vi "from string array.vi"(8 "error in (no error)":errorcluster, 9 "String Array":string[][](array[string]), 10 "version":string, 11 "module configuration in":refnum<class "Daqmx Module configuration.lvclass">) -> (0 "error out":errorcluster, 3 "module configuration out":refnum<class "Daqmx Module configuration.lvclass">)   [LabVIEW 2015, in "DAQmx Module Configuration.lvclass"]
uses:
  Daqmx Module configuration.lvclass
  Line.ctl
  <vilib>/NI/Tag Bus Module Framework/channel/TBM channel.lvclass
  Measurement Type.ctl
  Parameters.ctl
  <vilib>/NI/Tag Bus/tag/Data Type.ctl
  <vilib>/NI/Tag Bus Module Framework/channel/channel classification.ctl
  Daqmx Module configuration.lvclass/Daqmx Module configuration.ctl
  <vilib>/NI/Tag Bus/tag/tag descriptor.lvclass
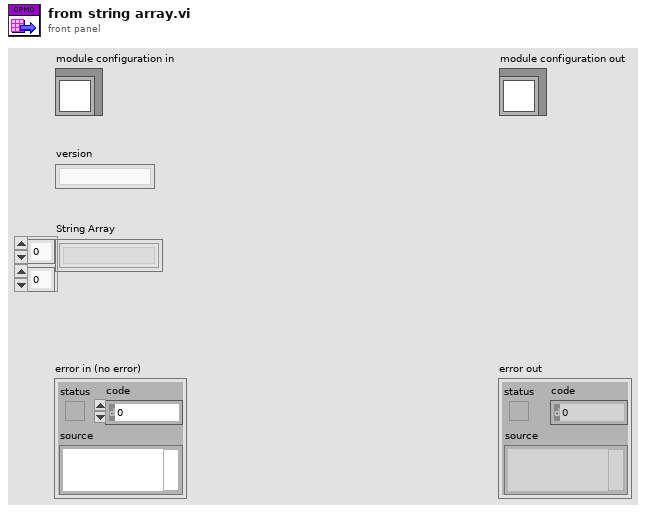
[diagram p1: front panel]
types:
  T1 = typedef "DAQmx Module Configuration.lvclass/Line.ctl" = cluster{"Channel Array":refnum<class "TBM channel.lvclass">[], "Physical Channel":string, "Measurement Type":T2, "Parameters":T3}
  T2 = typedef "DAQmx Module Configuration.lvclass/Measurement Type.ctl" = enum16{"Digital Input", "Digital Output", "Voltage Input", "Voltage Output", "Current Input", "Current Output", "RTD", "Thermocouple", "Strain", "PWM"}
  T3 = typedef "DAQmx Module Configuration.lvclass/Parameters.ctl" = cluster{"Digital Config":cluster{"Invert Lines?":bool}, "Voltage Config":cluster{"Maximum Value (V)":dbl, "Minimum Value (V)":dbl, "in terminal configuration (V)":i32, "out terminal configuration (V)":i32}, "Current Config":cluster{"Maximum Value (A)":dbl, "Minimum Value (A)":dbl, "shunt resistor location":i32, "input terminal configuration (C)":i32, "external shunt resistor value":dbl}, "RTD Config":cluster{"Maximum Value (°C)":dbl, "Minimum Value (°C)":dbl, "resistance configuration":i32, "r0":dbl, "current excitation value":dbl, "rtd type":i32, "current excitation source":i32}, "Thermocouple Config":cluster{"Minimum Value (C)":dbl, "Maximum Value (C)":dbl, "thermocouple type":i32, "cjc source":i32, "cjc value":dbl}, "Strain Config":cluster{"Maximum Value":dbl, "Minimum Value":dbl, "bridge information":cluster{"strain configuration":i32, "lead wire resistance":dbl, "initial bridge voltage":dbl, "voltage excitation source":i32, "voltage excitation value":dbl}, "strain gage information":cluster{"gage factor":dbl, "nominal gage resistance":dbl, "poisson ratio":dbl}}, "PWM Config":cluster{"Idle State":bool}}
  T4 = typedef "TBM channel.lvclass/channel classification.ctl" = enum16{"input data", "output data", "processing parameter", "processing result"}
  T5 = typedef "tag bus.lvlib/tag descriptor.lvclass/Data Type.ctl" = enum16{"Double", "Single", "I64", "I32", "I16", "I8", "U64", "U32", "U16", "U8", "Boolean", "String", "Array of Double", "Array of Single", "Array of I64", "Array of I32", "Array of I16", "Array of I8", "Array of U64", "Array of U32", "Array of U16", "Array of U8", "Array of Boolean", "Array of String"}
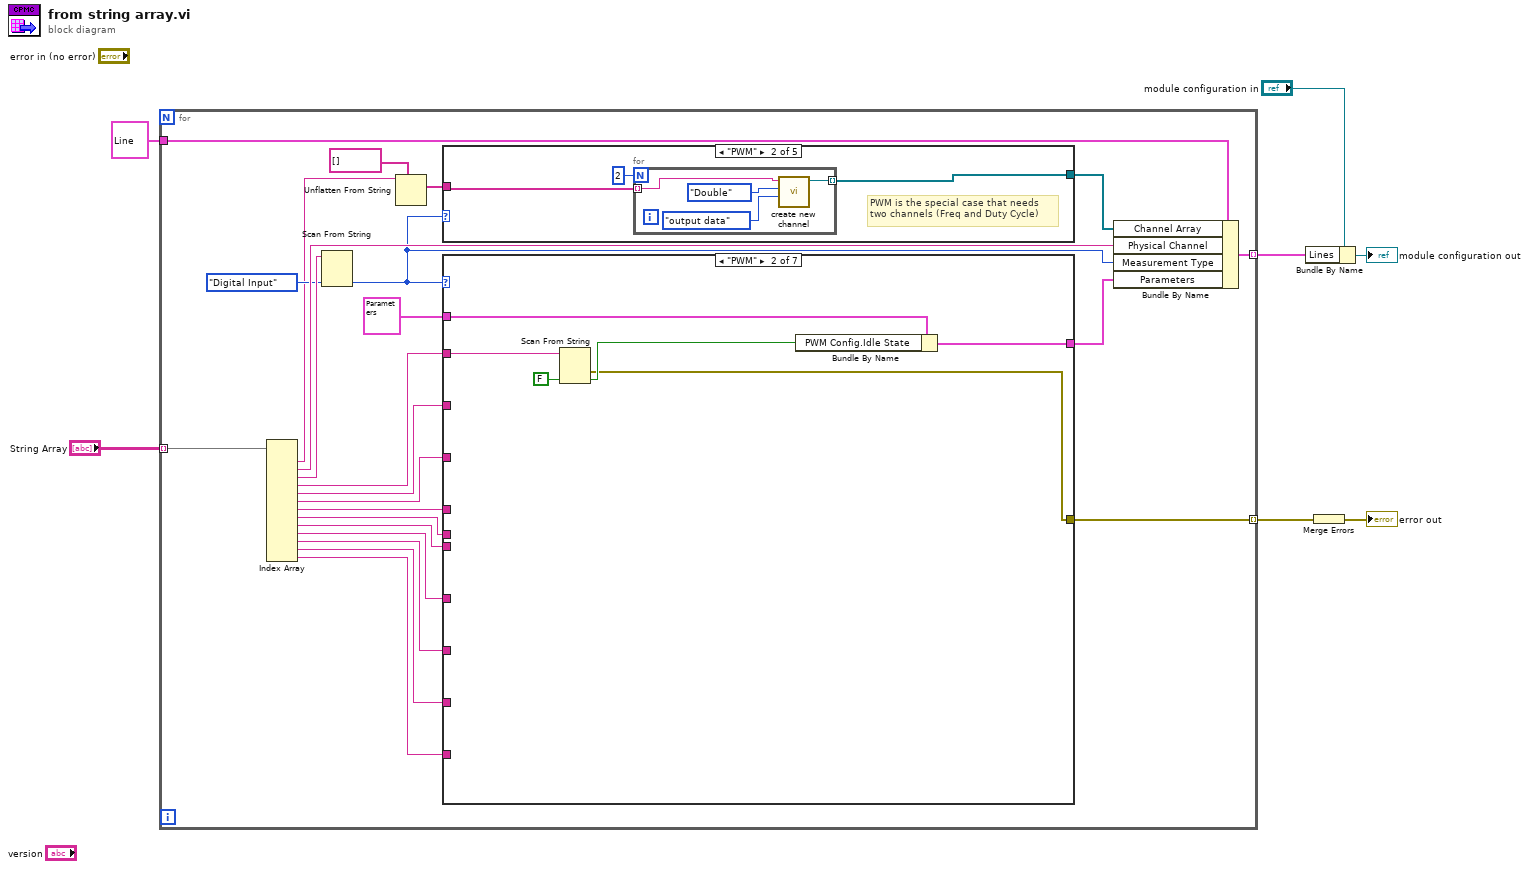
[diagram p0: block diagram]
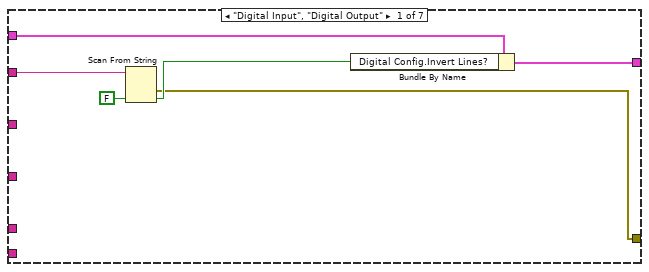
[diagram p2: hidden frame]
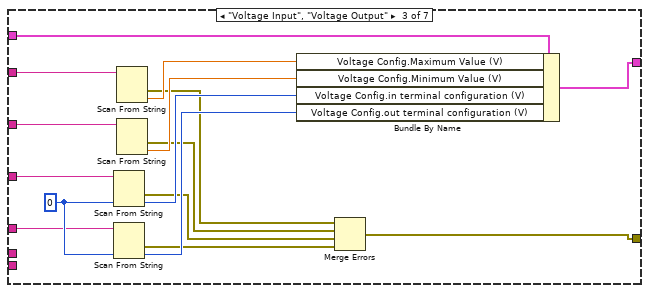
[diagram p3: hidden frame]
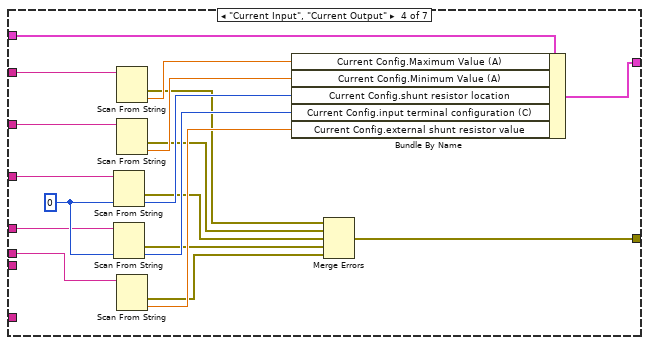
[diagram p4: hidden frame]
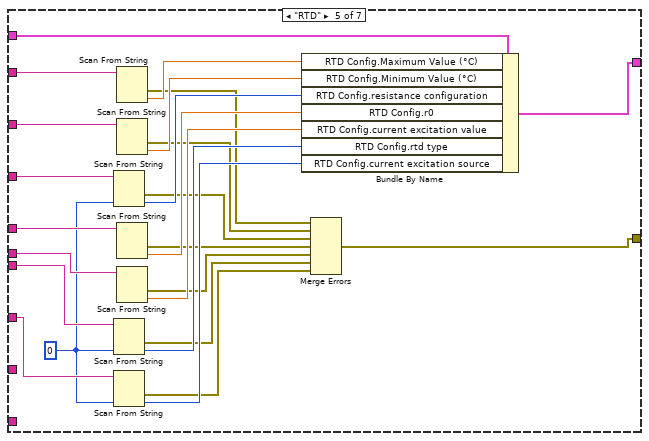
[diagram p5: hidden frame]
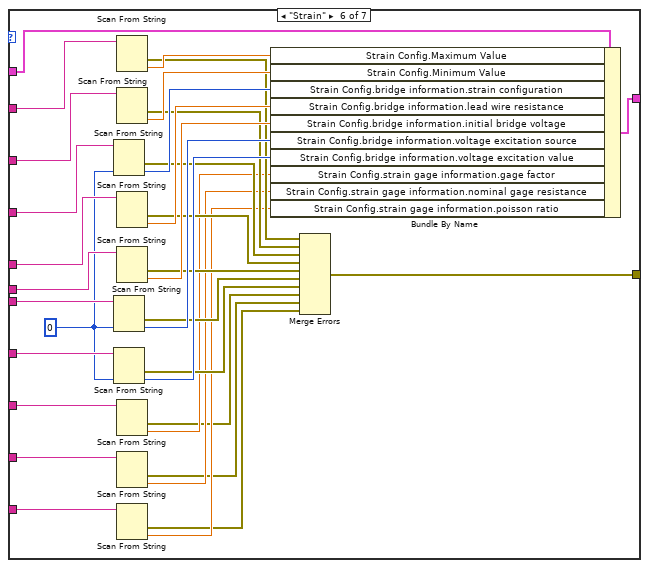
[diagram p6: hidden frame]
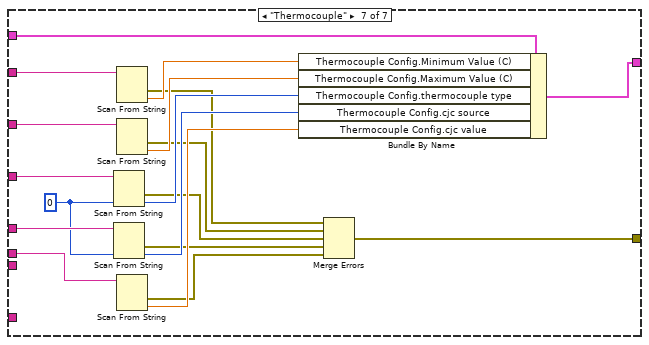
[diagram p7: hidden frame]
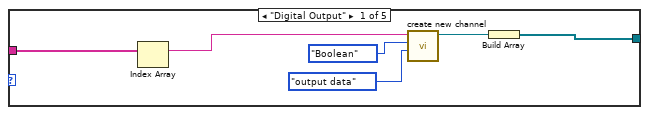
[diagram p8: hidden frame]
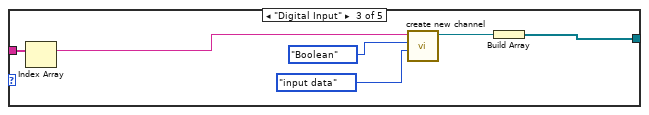
[diagram p9: hidden frame]
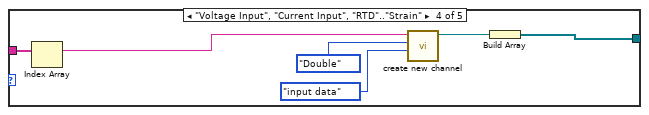
[diagram p10: hidden frame]
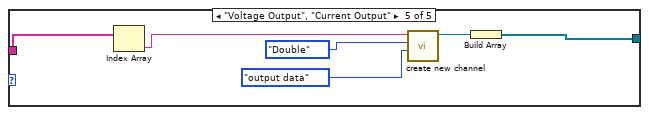
[diagram p11: hidden frame]
diagram:
  n1 = for {
    tunnel: "String Array" -> [w29] mode=indexing
    tunnel: T1 {"Channel Array"=[], "Physical Channel"="", "Measurement Type"=enum."Digital Input", "Parameters"={"Digital Config"={"Invert Lines?"=FALSE}, "Voltage Config"={"Maximum Value (V)"=5.0, "Minimum Value (V)"=-5.0, "in terminal configuration (V)"=-1, "out terminal configuration (V)"=-1}, "Current Config"={"Maximum Value (A)"=0.02, "Minimum Value (A)"=0.0, "shunt resistor location"=-1, "input terminal configuration (C)"=-1, "external shunt resistor value"=249.0}, "RTD Config"={"Maximum Value (°C)"=100.0, "Minimum Value (°C)"=0.0, "resistance configuration"=2, "r0"=100.0, "current excitation value"=0.0025, "rtd type"=10137, "current excitation source"=10167}, "Thermocouple Config"={"Minimum Value (C)"=0.0, "Maximum Value (C)"=100.0, "thermocouple type"=10072, "cjc source"=10116, "cjc value"=25.0}, "Strain Config"={"Maximum Value"=0.001, "Minimum Value"=-0.001, "bridge information"={"strain configuration"=10183, "lead wire resistance"=0.0, "initial bridge voltage"=0.0, "voltage excitation source"=10200, "voltage excitation value"=2.5}, "strain gage information"={"gage factor"=2.0, "nominal gage resistance"=350.0, "poisson ratio"=0.3}}, "PWM Config"={"Idle State"=FALSE}}} ("Line") -> [w31]
    tunnel: [w30] -> w4 mode=indexing
    tunnel: [w14] -> w2 mode=indexing
    n2 = Index Array(array=w29) -> (element #1=w9:string, element #2=w28:string, element #3=w27:string, element #4=w21:string, element #5=w20:string, element #6=w19:string, element #7=w18:string, element #8=w17:string, element #9=w16:string, element #10=w15:string, element #11=w13:string, element #12=w12:string, element #13=w11:string)  [unwired: 13 in]
    n3 = Scan From String(input string=w27, default 1=Measurement_Type."Digital Input" ("Measurement Type")) -> (output 1=w22:T2)  [unwired: 3 in, 3 out]
    n4 = Unflatten From String(type=string[] [], binary string=w9) -> (value=w8:string[])  [unwired: 3 in, 2 out]
    n5 = case shown="\"PWM\"" w22 {
      tunnel: w8 -> [w162 w164 w175 w181 w187]
      tunnel: [w158 w165 w171 w177 w183] -> w26
      frame "Digital Output" {
        n6 = Index Array(array=w162) -> (element=w157:string)  [unwired: 1 in]
        n7 = call <vilib>:"create new channel.vi"("channel classification"=channel_classification."output data", "data type"=Data_Type."Boolean", "channel name"=w157) -> ("channel"=w159:refnum<class "TBM channel.lvclass">)  [unwired: 8 in]
        n8 = Build Array(w159) -> (w158:refnum<class "TBM channel.lvclass">[])
      }
      frame "PWM" {
        # "PWM is the special case that needs\ntwo channels (Freq and Duty Cycle)"
        n9 = for {
          N: 2 -> [_]
          tunnel: [w167] -> w165 mode=indexing
          tunnel: w164 -> [w166] mode=indexing
          n10 = call <vilib>:"create new channel.vi"("channel classification"=channel_classification."output data", "data type"=Data_Type."Double", "channel name"=w166) -> ("channel"=w167:refnum<class "TBM channel.lvclass">)  [unwired: 8 in]
        }
      }
      frame "Digital Input" {
        n11 = Index Array(array=w175) -> (element=w170:string)  [unwired: 1 in]
        n12 = call <vilib>:"create new channel.vi"("channel classification"=channel_classification."input data", "data type"=Data_Type."Boolean", "channel name"=w170) -> ("channel"=w172:refnum<class "TBM channel.lvclass">)  [unwired: 8 in]
        n13 = Build Array(w172) -> (w171:refnum<class "TBM channel.lvclass">[])
      }
      frame "Voltage Input", "Current Input", "RTD".."Strain" {
        n14 = Index Array(array=w181) -> (element=w176:string)  [unwired: 1 in]
        n15 = call <vilib>:"create new channel.vi"("channel classification"=channel_classification."input data", "data type"=Data_Type."Double", "channel name"=w176) -> ("channel"=w178:refnum<class "TBM channel.lvclass">)  [unwired: 8 in]
        n16 = Build Array(w178) -> (w177:refnum<class "TBM channel.lvclass">[])
      }
      frame "Voltage Output", "Current Output" {
        n17 = Index Array(array=w187) -> (element=w182:string)  [unwired: 1 in]
        n18 = call <vilib>:"create new channel.vi"("channel classification"=channel_classification."output data", "data type"=Data_Type."Double", "channel name"=w182) -> ("channel"=w184:refnum<class "TBM channel.lvclass">)  [unwired: 8 in]
        n19 = Build Array(w184) -> (w183:refnum<class "TBM channel.lvclass">[])
      }
    }
    n20 = case shown="\"PWM\"" w22 {
      tunnel: T3 {"Digital Config"={"Invert Lines?"=FALSE}, "Voltage Config"={"Maximum Value (V)"=5.0, "Minimum Value (V)"=-5.0, "in terminal configuration (V)"=-1, "out terminal configuration (V)"=-1}, "Current Config"={"Maximum Value (A)"=0.02, "Minimum Value (A)"=0.0, "shunt resistor location"=-1, "input terminal configuration (C)"=-1, "external shunt resistor value"=249.0}, "RTD Config"={"Maximum Value (°C)"=100.0, "Minimum Value (°C)"=0.0, "resistance configuration"=2, "r0"=100.0, "current excitation value"=0.0025, "rtd type"=10137, "current excitation source"=10167}, "Thermocouple Config"={"Minimum Value (C)"=0.0, "Maximum Value (C)"=100.0, "thermocouple type"=10072, "cjc source"=10116, "cjc value"=25.0}, "Strain Config"={"Maximum Value"=0.001, "Minimum Value"=-0.001, "bridge information"={"strain configuration"=10183, "lead wire resistance"=0.0, "initial bridge voltage"=0.0, "voltage excitation source"=10200, "voltage excitation value"=2.5}, "strain gage information"={"gage factor"=2.0, "nominal gage resistance"=350.0, "poisson ratio"=0.3}}, "PWM Config"={"Idle State"=FALSE}} ("Parameters") -> [w37 w43 w59 w78 w103 w137 w156]
      tunnel: [w36 w42 w58 w77 w102 w136 w155] -> w23
      tunnel: w21 -> [w33 w39 w57 w76 w101 w135 w154]
      tunnel: w20 -> [_ _ w51 w70 w96 w130 w149]
      tunnel: w19 -> [_ _ w50 w69 w95 w129 w148]
      tunnel: w18 -> [_ _ w49 w68 w94 w128 w147]
      tunnel: w17 -> [_ _ _ w67 w93 w127 w146]
      tunnel: w16 -> [_ _ _ _ w89 w123 _]
      tunnel: w15 -> [_ _ _ _ w88 w122 _]
      tunnel: [w32 w38 w44 w60 w79 w113 w139] -> w14
      tunnel: w13 -> [_ _ _ _ _ w112 _]
      tunnel: w12 -> [_ _ _ _ _ w111 _]
      tunnel: w11 -> [_ _ _ _ _ w110 _]
      frame "Digital Input", "Digital Output" {
        n21 = Scan From String(input string=w33, default 1=FALSE ("Digital Config.Invert Lines?")) -> (error out=w32:errorcluster, output 1=w34:bool)  [unwired: 3 in, 2 out]
        n22 = Bundle By Name(cluster=w37, "Digital Config.Invert Lines?"=w34) -> (w36:T3)
      }
      frame "PWM" {
        n23 = Scan From String(input string=w39, default 1=FALSE ("Digital Config.Invert Lines?")) -> (error out=w38:errorcluster, output 1=w40:bool)  [unwired: 3 in, 2 out]
        n24 = Bundle By Name(cluster=w43, "PWM Config.Idle State"=w40) -> (w42:T3)
      }
      frame "Voltage Input", "Voltage Output" {
        w56 = 0 ("Voltage Config.out terminal configuration (V)")
        n25 = Scan From String(input string=w50, default 1=w56) -> (error out=w46:errorcluster, output 1=w54:i32)  [unwired: 3 in, 2 out]
        n26 = Scan From String(input string=w49, default 1=w56) -> (error out=w45:errorcluster, output 1=w55:i32)  [unwired: 3 in, 2 out]
        n27 = Scan From String(input string=w57) -> (error out=w48:errorcluster, output 1=w52:dbl)  [unwired: 4 in, 2 out]
        n28 = Scan From String(input string=w51) -> (error out=w47:errorcluster, output 1=w53:dbl)  [unwired: 4 in, 2 out]
        n29 = Bundle By Name(cluster=w59, "Voltage Config.Maximum Value (V)"=w52, "Voltage Config.Minimum Value (V)"=w53, "Voltage Config.in terminal configuration (V)"=w54, "Voltage Config.out terminal configuration (V)"=w55) -> (w58:T3)
        n30 = Merge Errors(w48, w47, w46, w45) -> (w44:errorcluster)
      }
      frame "Current Input", "Current Output" {
        w75 = 0 ("Voltage Config.out terminal configuration (V)")
        n31 = Scan From String(input string=w69, default 1=w75) -> (error out=w63:errorcluster, output 1=w73:i32)  [unwired: 3 in, 2 out]
        n32 = Scan From String(input string=w68, default 1=w75) -> (error out=w62:errorcluster, output 1=w74:i32)  [unwired: 3 in, 2 out]
        n33 = Scan From String(input string=w76) -> (error out=w65:errorcluster, output 1=w71:dbl)  [unwired: 4 in, 2 out]
        n34 = Scan From String(input string=w70) -> (error out=w64:errorcluster, output 1=w72:dbl)  [unwired: 4 in, 2 out]
        n35 = Scan From String(input string=w67) -> (error out=w61:errorcluster, output 1=w66:dbl)  [unwired: 4 in, 2 out]
        n36 = Bundle By Name(cluster=w78, "Current Config.Maximum Value (A)"=w71, "Current Config.Minimum Value (A)"=w72, "Current Config.shunt resistor location"=w73, "Current Config.input terminal configuration (C)"=w74, "Current Config.external shunt resistor value"=w66) -> (w77:T3)
        n37 = Merge Errors(w65, w64, w63, w62, w61) -> (w60:errorcluster)
      }
      frame "RTD" {
        w87 = 0 ("Voltage Config.out terminal configuration (V)")
        n38 = Scan From String(input string=w95, default 1=w87) -> (error out=w84:errorcluster, output 1=w99:i32)  [unwired: 3 in, 2 out]
        n39 = Scan From String(input string=w89, default 1=w87) -> (error out=w81:errorcluster, output 1=w91:i32)  [unwired: 3 in, 2 out]
        n40 = Scan From String(input string=w88, default 1=w87) -> (error out=w80:errorcluster, output 1=w90:i32)  [unwired: 3 in, 2 out]
        n41 = Scan From String(input string=w101) -> (error out=w86:errorcluster, output 1=w97:dbl)  [unwired: 4 in, 2 out]
        n42 = Scan From String(input string=w96) -> (error out=w85:errorcluster, output 1=w98:dbl)  [unwired: 4 in, 2 out]
        n43 = Scan From String(input string=w94) -> (error out=w83:errorcluster, output 1=w100:dbl)  [unwired: 4 in, 2 out]
        n44 = Scan From String(input string=w93) -> (error out=w82:errorcluster, output 1=w92:dbl)  [unwired: 4 in, 2 out]
        n45 = Bundle By Name(cluster=w103, "RTD Config.Maximum Value (°C)"=w97, "RTD Config.Minimum Value (°C)"=w98, "RTD Config.resistance configuration"=w99, "RTD Config.r0"=w100, "RTD Config.current excitation value"=w92, "RTD Config.rtd type"=w91, "RTD Config.current excitation source"=w90) -> (w102:T3)
        n46 = Merge Errors(w86, w85, w84, w83, w82, w81, w80) -> (w79:errorcluster)
      }
      frame "Strain" {
        w121 = 0 ("Voltage Config.out terminal configuration (V)")
        n47 = Scan From String(input string=w129, default 1=w121) -> (error out=w118:errorcluster, output 1=w133:i32)  [unwired: 3 in, 2 out]
        n48 = Scan From String(input string=w123, default 1=w121) -> (error out=w115:errorcluster, output 1=w125:i32)  [unwired: 3 in, 2 out]
        n49 = Scan From String(input string=w122, default 1=w121) -> (error out=w114:errorcluster, output 1=w124:i32)  [unwired: 3 in, 2 out]
        n50 = Scan From String(input string=w135) -> (error out=w120:errorcluster, output 1=w131:dbl)  [unwired: 4 in, 2 out]
        n51 = Scan From String(input string=w130) -> (error out=w119:errorcluster, output 1=w132:dbl)  [unwired: 4 in, 2 out]
        n52 = Scan From String(input string=w128) -> (error out=w117:errorcluster, output 1=w134:dbl)  [unwired: 4 in, 2 out]
        n53 = Scan From String(input string=w127) -> (error out=w116:errorcluster, output 1=w126:dbl)  [unwired: 4 in, 2 out]
        n54 = Scan From String(input string=w112) -> (error out=w106:errorcluster, output 1=w109:dbl)  [unwired: 4 in, 2 out]
        n55 = Scan From String(input string=w111) -> (error out=w105:errorcluster, output 1=w108:dbl)  [unwired: 4 in, 2 out]
        n56 = Scan From String(input string=w110) -> (error out=w104:errorcluster, output 1=w107:dbl)  [unwired: 4 in, 2 out]
        n57 = Bundle By Name(cluster=w137, "Strain Config.Maximum Value"=w131, "Strain Config.Minimum Value"=w132, "Strain Config.bridge information.strain configuration"=w133, "Strain Config.bridge information.lead wire resistance"=w134, "Strain Config.bridge information.initial bridge voltage"=w126, "Strain Config.bridge information.voltage excitation source"=w125, "Strain Config.bridge information.voltage excitation value"=w124, "Strain Config.strain gage information.gage factor"=w109, "Strain Config.strain gage information.nominal gage resistance"=w108, "Strain Config.strain gage information.poisson ratio"=w107) -> (w136:T3)
        n58 = Merge Errors(w120, w119, w118, w117, w116, w115, w114, w106, w105, w104) -> (w113:errorcluster)
      }
      frame "Thermocouple" {
        w138 = 0 ("Voltage Config.out terminal configuration (V)")
        n59 = Scan From String(input string=w148, default 1=w138) -> (error out=w142:errorcluster, output 1=w152:i32)  [unwired: 3 in, 2 out]
        n60 = Scan From String(input string=w147, default 1=w138) -> (error out=w141:errorcluster, output 1=w153:i32)  [unwired: 3 in, 2 out]
        n61 = Scan From String(input string=w154) -> (error out=w144:errorcluster, output 1=w150:dbl)  [unwired: 4 in, 2 out]
        n62 = Scan From String(input string=w149) -> (error out=w143:errorcluster, output 1=w151:dbl)  [unwired: 4 in, 2 out]
        n63 = Scan From String(input string=w146) -> (error out=w140:errorcluster, output 1=w145:dbl)  [unwired: 4 in, 2 out]
        n64 = Bundle By Name(cluster=w156, "Thermocouple Config.Minimum Value (C)"=w150, "Thermocouple Config.Maximum Value (C)"=w151, "Thermocouple Config.thermocouple type"=w152, "Thermocouple Config.cjc source"=w153, "Thermocouple Config.cjc value"=w145) -> (w155:T3)
        n65 = Merge Errors(w144, w143, w142, w141, w140) -> (w139:errorcluster)
      }
    }
    n66 = Bundle By Name(cluster=w31, "Channel Array"=w26, "Physical Channel"=w28, "Measurement Type"=w22, "Parameters"=w23) -> (w30:T1)
  }
  n67 = Bundle By Name(cluster="module configuration in", "Lines"=w4) -> (→"module configuration out":refnum<class "Daqmx Module configuration.lvclass">)
  n68 = Merge Errors(w2) -> (→"error out":errorcluster)
